vi "Generate Blend Points.vi"(6 "Index":i32, 8 "Speeds in":T2={"maxV (fps)"=20.0, "Accel Limit (fps^2)"=20.0, "Initial V (fps)"=0.0, "Sample Period (s)"=0.02, "Jerk Limit (fps^3)"=0.0, "Distances"=[]}, 9 "Initial Point":cluster{"x":dbl, "y":dbl, "th":dbl}={"x"=1.0, "y"=2.0, "th"=30.0}, 10 "Initial Acceleration":dbl format="%#_13g", 11 "Blend Info":T1) -> (0 "Speeds out":T2={"maxV (fps)"=20.0, "Accel Limit (fps^2)"=20.0, "Initial V (fps)"=0.0, "Sample Period (s)"=0.02, "Jerk Limit (fps^3)"=0.0, "Distances"=[]}, 3 "Trajectory Segment":T3, 5 "Final Acceleration":dbl)   [LabVIEW 2019]
uses:
  Speeds.ctl
  BlendType.ctl
panel:
  out "XY Graph":cluster{cluster{dbl, dbl}[]}[](graph)
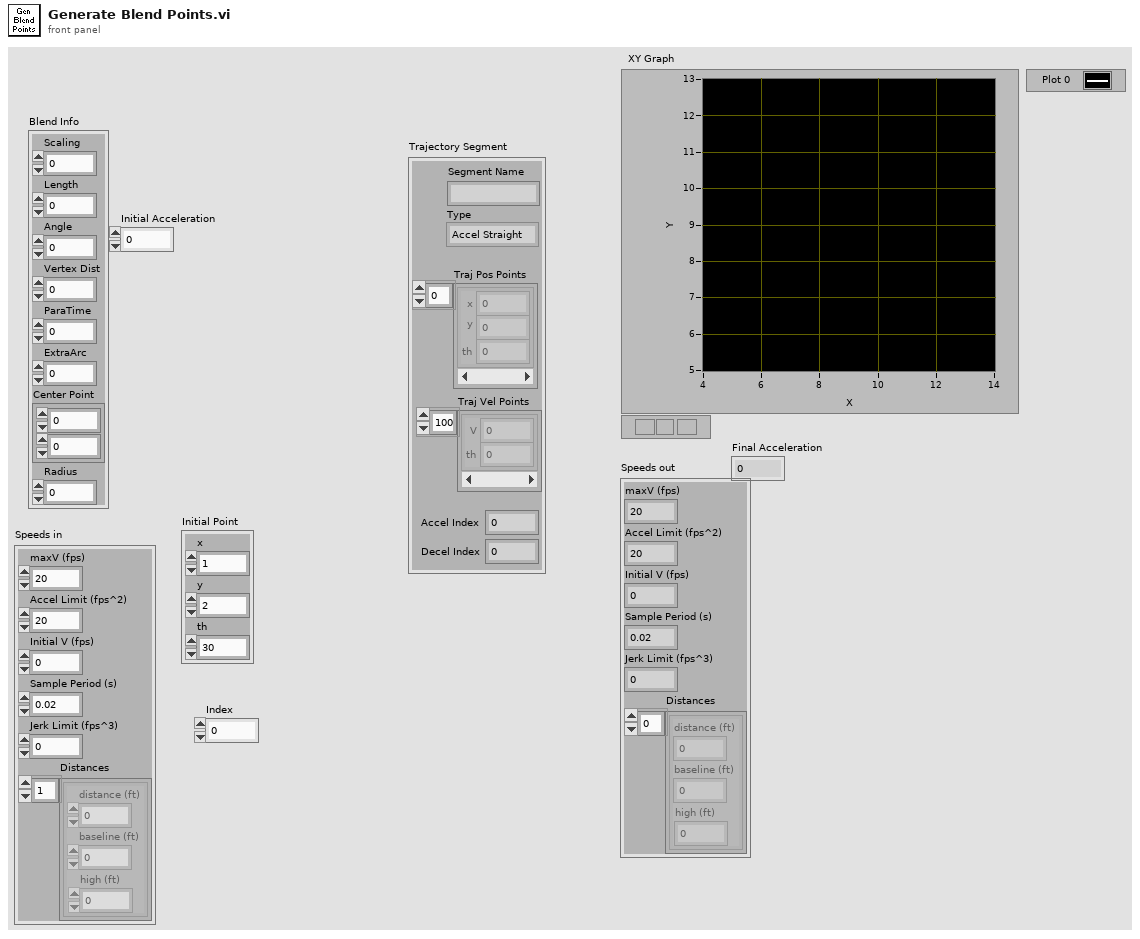
[diagram p1: front panel]
types:
  T1 = typedef "BlendType.ctl" = cluster{"Scaling":dbl, "Length":dbl, "Angle":dbl, "Vertex Dist":dbl, "ParaTime":dbl, "ExtraArc":dbl, "Center Point":cluster{dbl, dbl}, "Radius":dbl}
  T2 = typedef "Speeds.ctl" = cluster{"maxV (fps)":dbl, "Accel Limit (fps^2)":dbl, "Initial V (fps)":dbl, "Sample Period (s)":dbl, "Jerk Limit (fps^3)":dbl, "Distances":cluster{"distance (ft)":dbl, "baseline (ft)":dbl, "high (ft)":dbl}[]}
  T3 = cluster{"Segment Name":string, "Type":enum16{"Accel Straight", "Const Straight", "Blend", "Circle"}, "Traj Pos Points":cluster{"x":dbl, "y":dbl, "th":dbl}[], "Traj Vel Points":cluster{"V":dbl, "th":dbl}[], "Accel Index":i32, "Decel Index":i32}
  T4 = enum16{"Accel Straight", "Const Straight", "Blend", "Circle"}
  T5 = cluster{string, "Type":enum16{"Accel Straight", "Const Straight", "Blend", "Circle"}, cluster{dbl, dbl, dbl}[], cluster{dbl, dbl}[], "Accel Index":i32, "Decel Index":i32}
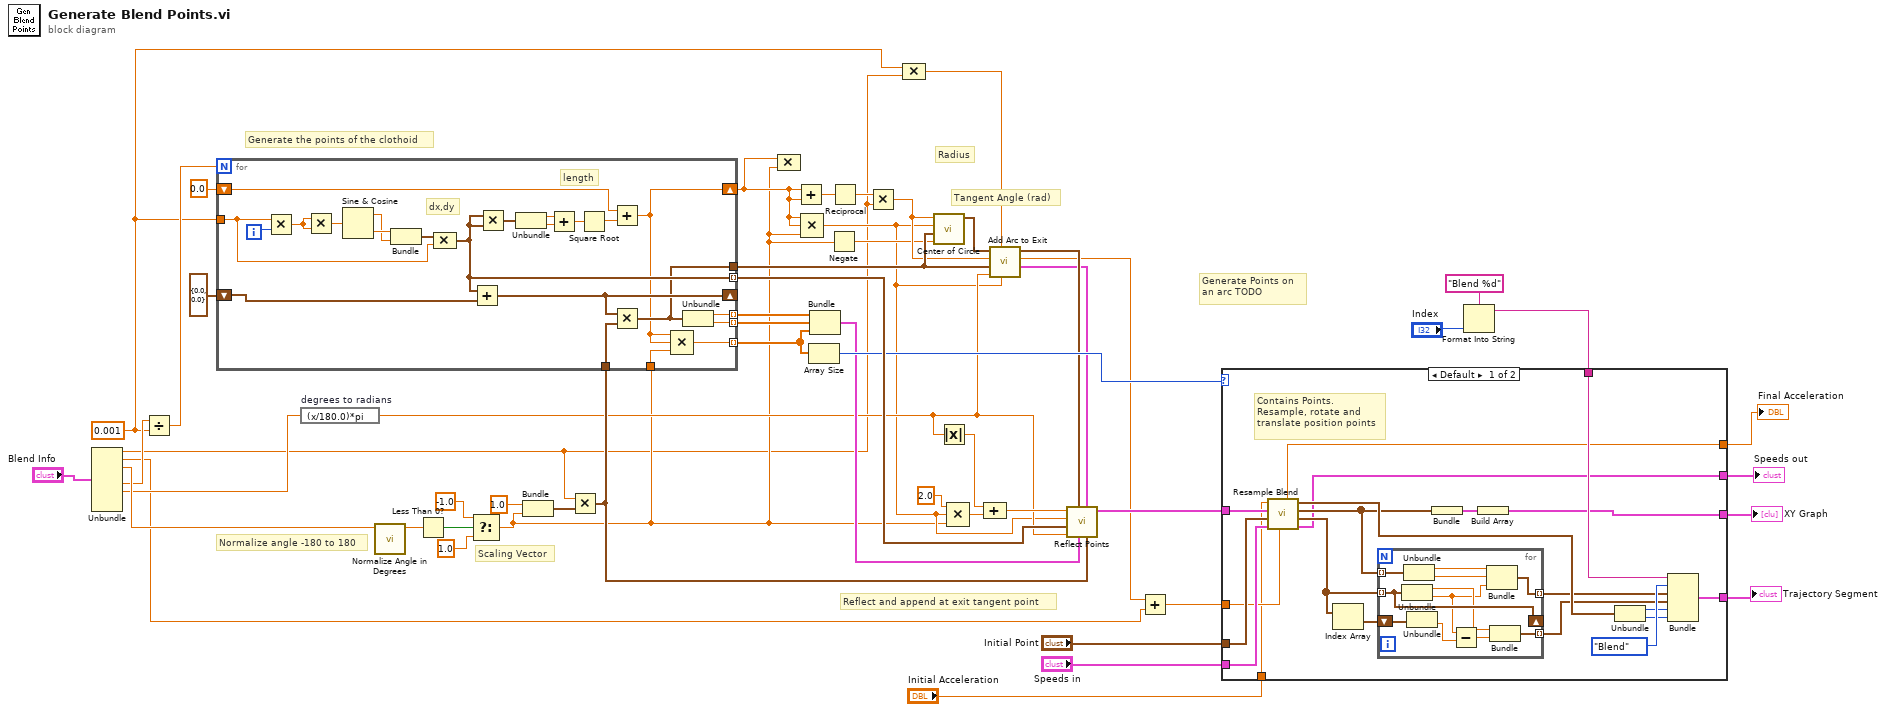
[diagram p0: block diagram]
diagram:
  w4 = 0.001
  # "Generate Points on \nan arc TODO"
  # "Reflect and append at exit tangent point"
  # "Scaling Vector"
  # "Normalize angle -180 to 180"
  # "Radius"
  # "Tangent Angle (rad)"
  # "Generate the points of the clothoid"
  n1 = Unbundle("Blend Info") -> ("Scaling"=w1:dbl, "Length"=w8:dbl, "Angle"=w23:dbl, "ParaTime"=w22:dbl, "ExtraArc"=w17:dbl)  [unwired: 3 out]
  n2 = Divide(x=w22, y=w4) -> (x/y=w6:dbl)
  n3 = expression code="(x/180.0)*pi" "degrees to radians"(w17) -> (w13:dbl)
  n4 = call "Normalize Angle in Degrees.vi"("Angle deg"=w23) -> ("Angle"=w34:dbl)  [unwired: 10 in]
  n5 = Less Than 0?(x=w34) -> (x < 0?=w37:bool)
  n6 = Select(t=-1.0, s=w37, f=1.0) -> (s? t:f=w2:dbl)
  n7 = Bundle(1.0, w2) -> (w35:cluster{dbl, dbl})  [unwired: 1 in]
  n8 = Multiply(x=w1, y=w35) -> (x*y=w15:cluster{dbl, dbl})
  n9 = for {
    N: w6 -> [_]
    shift-right: [w69] -> _
    shift-left: cluster{dbl, dbl} {0.0, 0.0} -> [w71]
    tunnel: w4 -> [w68]
    shift-right: [w58] -> w5
    shift-left: 0.0 -> [w63]
    tunnel: [w59] -> w48
    tunnel: [w61] -> w52 mode=indexing
    tunnel: w15 -> [w60]
    tunnel: [w55] -> w32 mode=indexing
    tunnel: [w54] -> w33 mode=indexing
    tunnel: w2 -> [w57]
    tunnel: [w56] -> w30 mode=indexing
    i -> [w76]
    # "length"
    # "dx,dy"
    n10 = Multiply(x=w68, y=w76) -> (x*y=w70:dbl)
    n11 = Multiply(x=w70, y=w70) -> (x*y=w75:dbl)
    n12 = Sine & Cosine(0:w75) -> (1:w73:dbl, 2:w74:dbl)
    n13 = Bundle(w74, w73) -> (w72:cluster{dbl, dbl})  [unwired: 1 in]
    n14 = Compound Arithmetic op=MULTIPLY(w72, w68) -> (w61:cluster{dbl, dbl})
    n15 = Add(x=w61, y=w71) -> (x+y=w69:cluster{dbl, dbl})
    n16 = Multiply(x=w61, y=w61) -> (x*y=w67:cluster{dbl, dbl})
    n17 = Unbundle(w67) -> (w66:dbl, w65:dbl)
    n18 = Add(x=w66, y=w65) -> (x+y=w64:dbl)
    n19 = Square Root(x=w64) -> (sqrt(x)=w62:dbl)
    n20 = Add(x=w63, y=w62) -> (x+y=w58:dbl)
    n21 = Multiply(x=w69, y=w60) -> (x*y=w59:cluster{dbl, dbl})
    n22 = Compound Arithmetic op=MULTIPLY(w58, w58, w57) -> (w56:dbl)
    n23 = Unbundle(w59) -> (w55:dbl, w54:dbl)
  }
  n24 = Compound Arithmetic op=MULTIPLY(w5, w2) -> ()  [unwired: 1 out]
  n25 = Add(x=w5, y=w5) -> (x+y=w51:dbl)
  n26 = Compound Arithmetic op=MULTIPLY(w5, w5, w2) -> (w10:dbl)
  n27 = Array Size(array=w30) -> (size(s)=w41:i32)
  n28 = Bundle(w32, w33, w30) -> (w31:cluster{dbl[], dbl[], dbl[]})  [unwired: 1 in]
  n29 = Negate(x=w2) -> (-x=w18:dbl)
  n30 = Reciprocal(x=w51) -> (1/x=w50:dbl)
  n31 = Multiply(x=w50, y=w1) -> (x*y=w47:dbl)
  n32 = Compound Arithmetic op=MULTIPLY(w4, w1) -> (w3:dbl)
  n33 = call "Center of Circle.vi"("Sign"=w18, "Tangent Point"=w48, "Tangent Angle"=w10, "Radius"=w47) -> ("Center Point"=w49:cluster{dbl, dbl})  [unwired: 7 in]
  n34 = Absolute Value(x=w13) -> (abs(x)=w16:dbl)
  n35 = Compound Arithmetic op=MULTIPLY(2.0, w10, w2) -> (w25:dbl)
  n36 = Compound Arithmetic op=ADD(w16, w25) -> (w26:dbl)
  n37 = call "Add Arc to Exit.vi"("Tangent Start Angle (rad)"=w10, "Dist per Points"=w3, "Additional circle arc (rad)"=w13, "Tangent Point"=w48, "Radius"=w47, "Center Point"=w49) -> ("Point Arrays"=w14:cluster{dbl[], dbl[], dbl[]}, "Arc Distance"=w9:dbl, "Blend Exit Point"=w28:cluster{dbl, dbl})  [unwired: 3 in]
  n38 = call "Reflect Points.vi"("Scaling Vector"=w15, "Arc Point Arrays"=w14, "Blend Point Arrays"=w31, "Blend Exit Point"=w28, "Extra Arc rad"=w13, "Delta Points"=w52, "Tangent Angle (rad)"=w10, "Angle"=w26) -> ("Point Arrays"=w29:cluster{dbl[], dbl[], dbl[]})  [unwired: 3 in]
  n39 = Add(x=w9, y=w8) -> (x+y=w7:dbl)
  n40 = Format Into String(format string="Blend %d", "Index") -> (resulting string=w21:string)  [unwired: 2 in, 1 out]
  n41 = case shown="Default" w41 {
    tunnel: "Initial Point" -> [w92 _]
    tunnel: [w95 _] -> w44
    tunnel: "Speeds in" -> [w90 w108]
    tunnel: w21 -> [w94 _]
    tunnel: [w93 _] -> w42
    tunnel: [w80 w108] -> w40
    tunnel: w29 -> [w79 _]
    tunnel: w7 -> [w89 _]
    tunnel: "Initial Acceleration" -> [w78 _]
    tunnel: [w77 _] -> w11
    frame Default {
      # "Contains Points.\nResample, rotate and\ntranslate position points"
      n42 = call "Resample Blend.vi"("Length"=w89, "Speeds in"=w90, "Initial Point"=w92, "Point Arrays"=w79, "Initial Acceleration"=w78) -> ("Speeds out"=w80:T2, "Vel Points"=w81:cluster{dbl, dbl}[], "Points"=w82:cluster{dbl, dbl}[], "Indices"=w88:cluster{"Accel Index":i32, "Decel Index":i32}, "Final Acceleration"=w77:dbl)  [unwired: 2 in]
      n43 = Index Array(array=w81) -> (element=w85:cluster{dbl, dbl})  [unwired: 1 in]
      n44 = for {
        tunnel: w82 -> [w107] mode=indexing
        tunnel: [w104] -> w83 mode=indexing
        tunnel: w81 -> [w100] mode=indexing
        shift-right: [w100] -> _
        shift-left: w85 -> [w102]
        tunnel: [w97] -> w84 mode=indexing
        n45 = Unbundle(w100) -> (w99:dbl, w98:dbl)
        n46 = Unbundle(w107) -> (w106:dbl, w105:dbl)
        n47 = Unbundle(w102) -> (w103:dbl)  [unwired: 1 out]
        n48 = Subtract(x=w98, y=w103) -> (x-y=w101:dbl)
        n49 = Bundle(w106, w105, w98) -> (w104:cluster{dbl, dbl, dbl})  [unwired: 1 in]
        n50 = Bundle(w99, w101) -> (w97:cluster{dbl, dbl})  [unwired: 1 in]
      }
      n51 = Bundle("Points"=w82) -> (w96:cluster{"Points":cluster{dbl, dbl}[]})  [unwired: 1 in]
      n52 = Build Array(w96) -> (w93:cluster{"Points":cluster{dbl, dbl}[]}[])
      n53 = Unbundle(w88) -> ("Accel Index"=w87:i32, "Decel Index"=w86:i32)
      n54 = Bundle(w94, "Type"=T4."Blend", w83, w84, "Accel Index"=w87, "Decel Index"=w86) -> (w95:T5)  [unwired: 1 in]
    }
    frame 0 {
    }
  }
  "Trajectory Segment" <- w44
  "XY Graph" <- w42
  "Speeds out" <- w40
  "Final Acceleration" <- w11
